vi "Format Data to File.vi"(8 "error in":errorcluster, 10 "Time Format String (%c)":string="%H:%M:%S%2u", 11 "Data In":dbl[](array[numeric])) -> (0 "error out":errorcluster, 3 "Spreadsheet String Out":string)   [LabVIEW 2021]
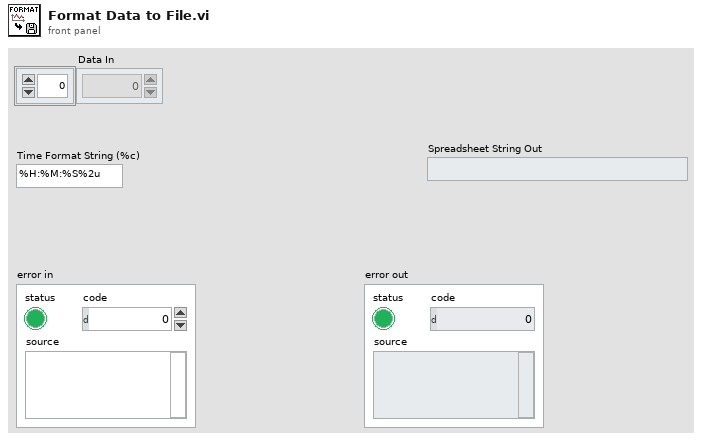
[diagram p1: front panel]
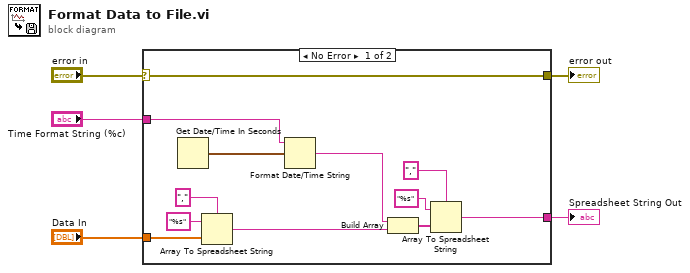
[diagram p0: block diagram]
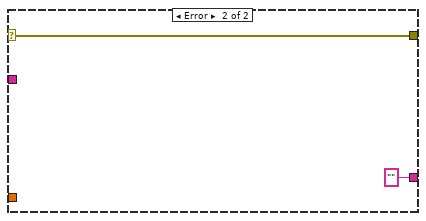
[diagram p2: hidden frame]
diagram:
  n1 = case shown="No Error" "error in" {
    selector: "error in" -> [w17 w19]
    tunnel: [w17 w19] -> w4
    tunnel: "Data In" -> [w16 _]
    tunnel: "Time Format String (%c)" -> [w10 _]
    tunnel: [w6 "" ("spreadsheet string")] -> w1
    frame No Error {
      n2 = Get Date/Time In Seconds() -> (seconds since 1Jan1904=w11:timestamp)
      n3 = Array To Spreadsheet String(delimiter (Tab)=",", array=w16, 3:"%s" ("format string")) -> (spreadsheet string=w9:string)
      n4 = Format Date/Time String(time format string (%c)=w10, seconds (now)=w11) -> (date/time string=w8:string)  [unwired: 1 in]
      n5 = Build Array(w8, w9) -> (w7:string[])
      n6 = Array To Spreadsheet String(delimiter (Tab)=",", array=w7, 3:"%s" ("format string")) -> (spreadsheet string=w6:string)
    }
    frame Error {
    }
  }
  "error out" <- w4
  "Spreadsheet String Out" <- w1
